vi "Find All NI-SWITCH Custom Devices.vi"(8 "error in":errorcluster, 11 "target in":refnum<k24>) -> (0 "error out":errorcluster, 2 "ni-switch custom devices":T1[](array[typedef]) format="%.0x", 3 "target out":refnum<k24>)   [LabVIEW 2019, in "NI-SWITCH Scripting.lvlib"]
doc: "Returns all NI-SWITCH custom devices under the specified target."
uses:
  NI-SWITCH Scripting.lvlib
  NationalInstruments.VeriStand.SystemDefinitionAPI
  <vilib>/NI VeriStand/Custom Device API/Custom Device Item Ref.ctl
  Shared/Constants.vi
  Shared/NI-SWITCH Shared.lvlib
  <vilib>/NI VeriStand/Custom Device API/Custom Device API.lvlib
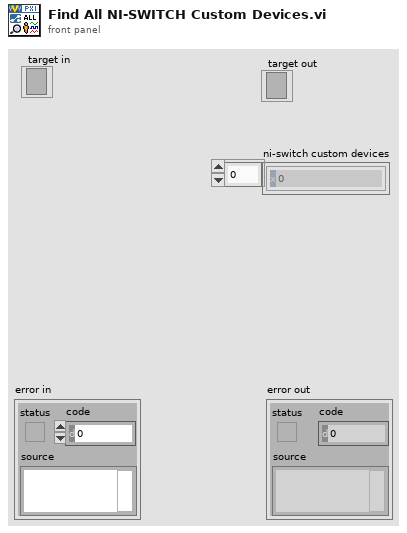
[diagram p1: front panel]
types:
  T1 = typedef "Custom Device API.lvlib/Custom Device Item Ref.ctl" = u64
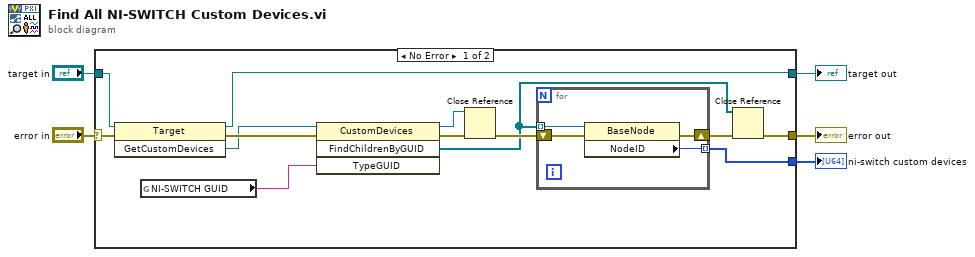
[diagram p0: block diagram]
diagram:
  n1 = case shown="No Error" "error in" {
    selector: "error in" -> [w18 w24]
    tunnel: [w9 w24] -> w5
    tunnel: "target in" -> [w17 w23]
    tunnel: [w11 w23] -> w2
    tunnel: [w10 _] -> w1
    frame No Error {
      n2 = invoke class="Target" method="GetCustomDevices"(reference=w17, error in=w18) -> (reference out=w11:refnum<k24>, error out=w16:errorcluster, "GetCustomDevices"=w15:refnum<k24>)  [unwired: 1 in]
      n3 = global read "Constants.vi" "NI-SWITCH GUID"() -> (w7:string)
      n4 = invoke class="CustomDevices" method="FindChildrenByGUID"(reference=w15, error in=w16, "TypeGUID"=w7) -> (reference out=w14:refnum<k24>, error out=w13:errorcluster, "FindChildrenByGUID"=w6:refnum<k24>[])  [unwired: 1 in, 1 out]
      n5 = Close Reference(reference=w14, error in (no error)=w13) -> (error out=w12:errorcluster)
      n6 = for {
        tunnel: [w21] -> w10 mode=indexing
        shift-right: [w20] -> w8
        shift-left: w12 -> [w22]
        tunnel: w6 -> [w19] mode=indexing
        n7 = property class="BaseNode"(reference=w19, error in=w22) -> (error out=w20:errorcluster, "NodeID"=w21:u64)  [unwired: 1 out]
      }
      n8 = Close Reference(reference=w6, error in (no error)=w8) -> (error out=w9:errorcluster)
    }
    frame Error {
    }
  }
  "target out" <- w2
  "error out" <- w5
  "ni-switch custom devices" <- w1
